vi "Get Registers.vi"(0 "Out Divider":i32=1, 1 "PllCntrl":T1={"PLL PWR"=3, "MUX out"=0, "Phase"=1, "Low Noise"=TRUE, "REF X2"=FALSE, "Mute till LD"=TRUE, "Icp"=15, "Band Sel Div"=100, "REF Divide"=5, "Reference(MHz)"=10.0} {"Icp" scale=0.0..15.0; "MUX out" items=["3-State", "GND", "Vcc", "Analog LD", "Digital LD", "REF / R", "RF / N"]; "PLL PWR" scale=0.0..3.0}, 3 "RF out EN":bool=TRUE, 4 "Power Down":bool, 15 "INT":i16, 16 "FRAC":i32, 17 "MOD":i32) -> (14 "concatenated string":string, 19 "Allregout":u32[](array[numeric])=[4194309, 10896444, 1203, 97986, 134254497, 65536000] format="%08x")   [LabVIEW 2012]
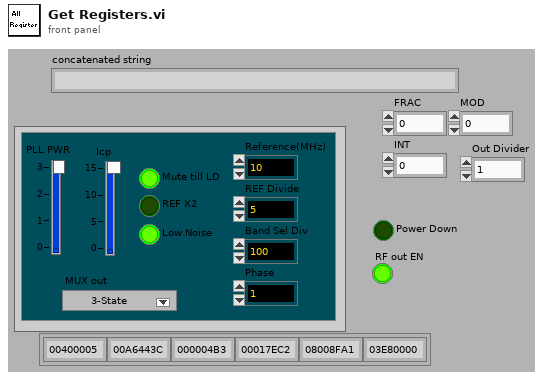
[diagram p1: front panel]
types:
  T1 = cluster{"PLL PWR":i8, "MUX out":u16, "Phase":i16, "Low Noise":bool, "REF X2":bool, "Mute till LD":bool, "Icp":i32, "Band Sel Div":i32, "REF Divide":i16, "Reference(MHz)":dbl}
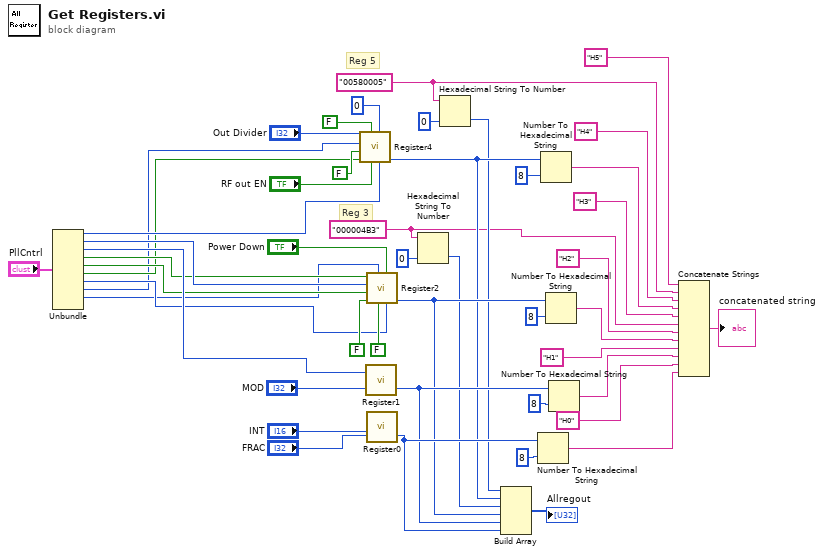
[diagram p0: block diagram]
diagram:
  w2 = "000004B3"
  w6 = "00580005"
  # "Reg 3"
  # "Reg 5"
  n1 = Unbundle("PllCntrl") -> ("PLL PWR"=w35:i8, "MUX out"=w34:u16, "Phase"=w33:i16, "Low Noise"=w32:bool, "REF X2"=w31:bool, "Mute till LD"=w30:bool, "Icp"=w29:i32, "Band Sel Div"=w28:i32, "REF Divide"=w27:i16)  [unwired: 1 out]
  n2 = call "Register4.vi"("RF Out PWR"=w35, "Aux Out PWR"=i8 0, "RF out EN"="RF out EN", "AUX OUT EN"=FALSE, "Mute till LD"=w30, "AUX OUT SEL"=FALSE, "Band Sel Div"=w28, "Out Divider"="Out Divider") -> ("HEX4"=w7:u32)  [unwired: 3 out]
  n3 = call "Register1.vi"("MOD"="MOD", "Phase"=w33) -> ("HEX1"=w9:u32)  [unwired: 1 out]
  n4 = call "Register2.vi"("Icp"=w29, "Power Down"="Power Down", "Double Buff"=FALSE, "REF Divide"=w27, "REF /2"=FALSE, "REF X2"=w31, "MUX out"=w34, "Low Noise"=w32) -> ("HEX2"=w8:u32)  [unwired: 3 out]
  n5 = call "Register0.vi"("FRAC"="FRAC", "INT"="INT") -> ("HEX0"=w10:u32)  [unwired: 1 out]
  n6 = Hexadecimal String To Number(string=w2, default (0uL)=u32 0 ("default (0 U32)")) -> (number=w1:u32)  [unwired: 1 in, 1 out]
  n7 = Hexadecimal String To Number(string=w6, default (0uL)=u32 0 ("default (0 U32)")) -> (number=w4:u32)  [unwired: 1 in, 1 out]
  n8 = Build Array(w4, w7, w1, w8, w9, w10) -> (→"Allregout":u32[])
  n9 = Number To Hexadecimal String(1:i16 8 ("width (-)"), 2:w10) -> (0:w13:string)
  n10 = Number To Hexadecimal String(1:i16 8 ("width (-)"), 2:w7) -> (0:w20:string)
  n11 = Number To Hexadecimal String(1:i16 8 ("width (-)"), 2:w8) -> (0:w17:string)
  n12 = Number To Hexadecimal String(1:i16 8 ("width (-)"), 2:w9) -> (0:w15:string)
  n13 = Concatenate Strings("H5", w6, "H4", w20, "H3", w2, "H2", w17, "H1", w15, "H0", w13) -> (→"concatenated string":string)
